vi "GenerateIP'stoPing.vi"(10 "Gateway":string, 11 "Subnet Mask":string) -> (3 "subarray":string[](array[string]))   [LabVIEW 2013]
panel:
  out "Array":string[][](array[string])
  out "reversed":string
  out "array":string[](array[string])
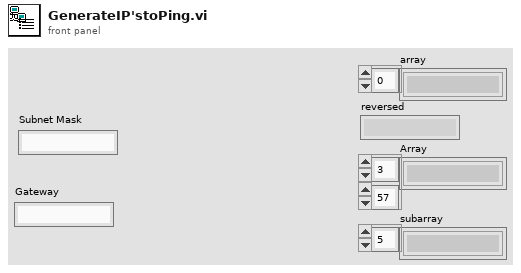
[diagram p1: front panel]
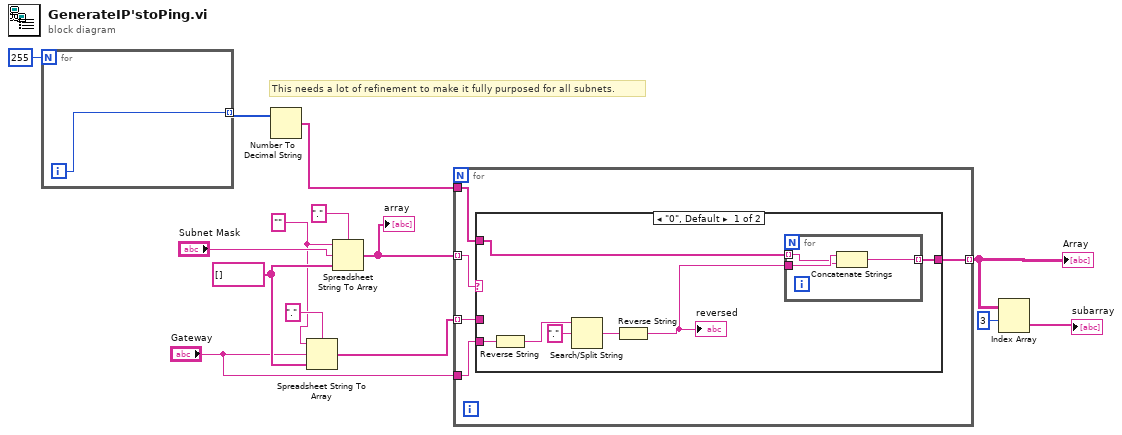
[diagram p0: block diagram]
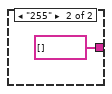
[diagram p2: hidden frame]
diagram:
  w10 = string[] []
  w8 = "" ("format string")
  # "This needs a lot of refinement to make it fully purposed for all subnets."
  n1 = for {
    N: 255 -> [_]
    tunnel: [w15] -> w5 mode=indexing
    i -> [w15]
  }
  n2 = Number To Decimal String(number=w5) -> (decimal integer string=w4:string[])  [unwired: 1 in]
  n3 = Spreadsheet String To Array(delimiter (Tab)=".", format string=w8, spreadsheet string="Gateway", array type (2D Dbl)=w10) -> (array=w9:string[])
  n4 = Spreadsheet String To Array(delimiter (Tab)=".", format string=w8, spreadsheet string="Subnet Mask", array type (2D Dbl)=w10) -> (array=w12:string[])
  "array" <- w12
  n5 = for {
    tunnel: w12 -> [w20] mode=indexing
    tunnel: w9 -> [w19] mode=indexing
    tunnel: "Gateway" -> [w18]
    tunnel: w4 -> [w17]
    tunnel: [w16] -> w3 mode=indexing
    n6 = case shown="\"0\", Default" w20 {
      tunnel: w19 -> [_ _]
      tunnel: w18 -> [w27 _]
      tunnel: w17 -> [w23 _]
      tunnel: [w21 string[] []] -> w16
      frame "0", Default {
        n7 = Reverse String(1:w27) -> (0:w26:string)
        n8 = Search/Split String(string=w26, search string/char (-)=".") -> (match + rest of string=w24:string)  [unwired: 1 in, 2 out]
        n9 = Reverse String(1:w24) -> (0:w22:string)
        "reversed" <- w22
        n10 = for {
          tunnel: w23 -> [w29] mode=indexing
          tunnel: w22 -> [w30]
          tunnel: [w28] -> w21 mode=indexing
          n11 = Concatenate Strings(w30, w29) -> (w28:string)
        }
      }
      frame "255" {
      }
    }
  }
  "Array" <- w3
  n12 = Index Array(array=w3, index (row)=3) -> (element=→"subarray":string[])  [unwired: 1 in]
